vi "CODMn通讯.vi"() -> ()   [LabVIEW 2016, in "斯坦道CODMn.lvlib"]
uses:
  <vilib>/NI/Modbus Library/API/Wrapper/Create TCP Slave.vi
  <vilib>/NI/Modbus Library/API/slave/Modbus Slave.lvclass
  <vilib>/Plasmionique/MB Master/MB_Master/MB_Master.lvclass
  <vilib>/Plasmionique/MB Master/MB Master.lvlib
  <vilib>/Utility/config.llb/NI_LVConfig.lvlib
  <vilib>/NI/Modbus Library/API/Wrapper/API Main.lvlib
panel:
  in  "读取数据":bool
  in  "释放串口":bool
  in  "打开串口":bool
  out "队列中元素数量":i32
  out "元素":cluster{"命令":string}[](array[cluster])
  out "待处理插入数量":i32
  out "读取公式":u16[](array[numeric])
  out "读取参数":u16[](array[numeric])
  out "数据存储":u16[](array[numeric])
  out "温度":bool[](array[boolean])
  out "M输出点":bool[](array[boolean])
  out "ORP、时间":u16[](array[numeric])
  out "测量状态":u16[](array[numeric])
  out "通讯状态":bool
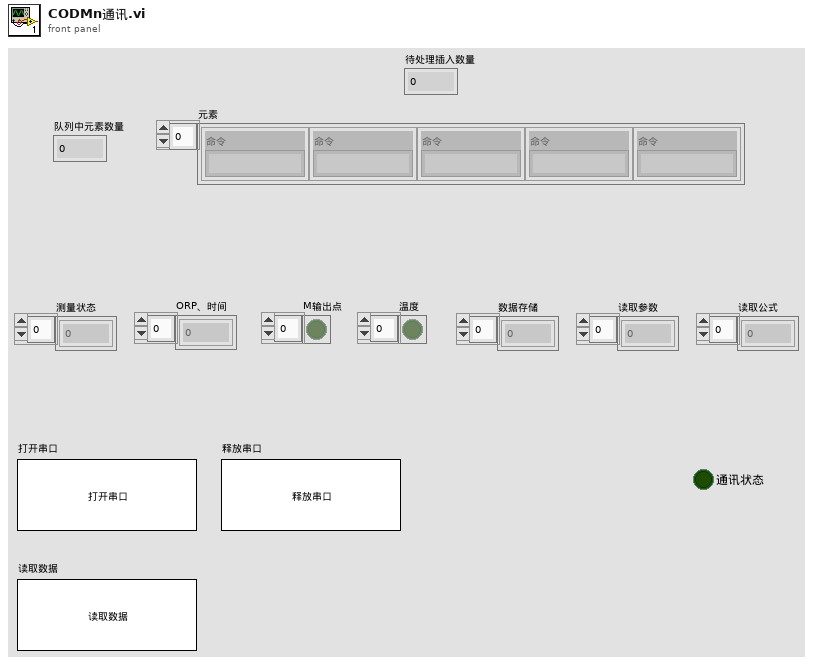
[diagram p1: front panel]
types:
  T1 = typedef "NI_LVConfig.lvlib/Config Data RefNum.ctl" = refnum<k1>
  T2 = enum16{"空闲", "水样测试", "标样核查", "零点核查", "跨度核查", "空白测试", "平行样测试", "质控样", "空白校准", "标样校准", "加标回收"}
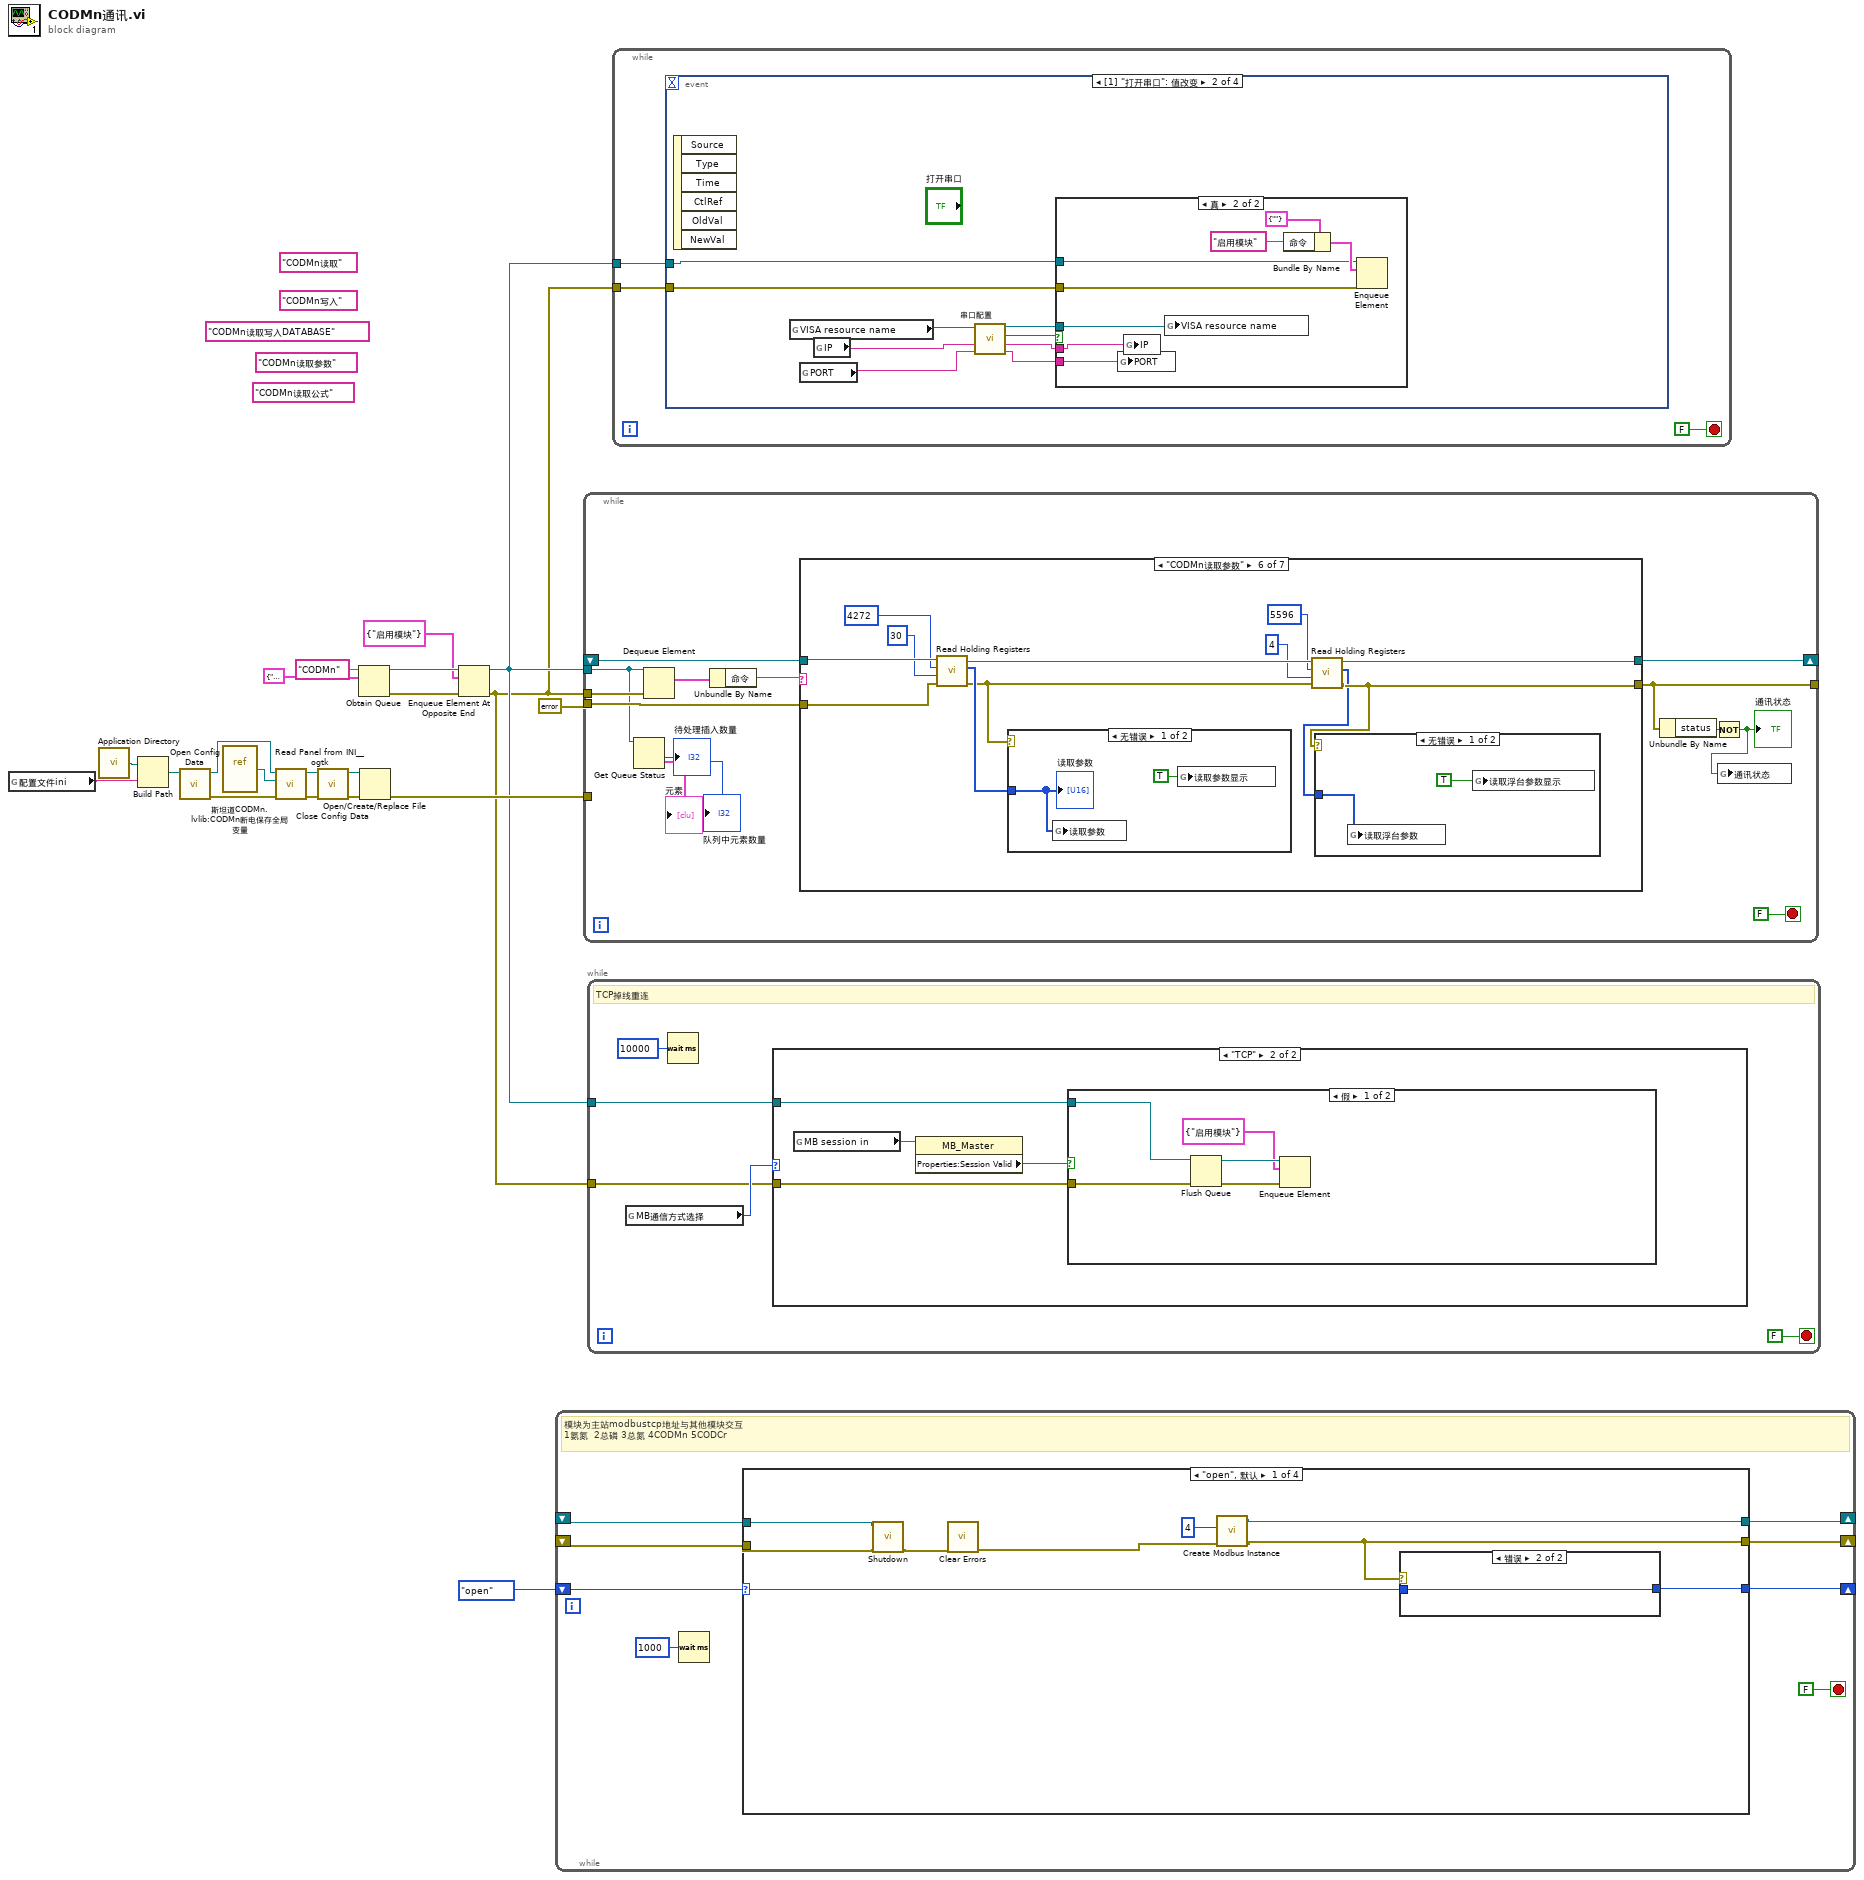
[diagram p0: block diagram]
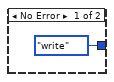
[diagram p4: hidden frame]
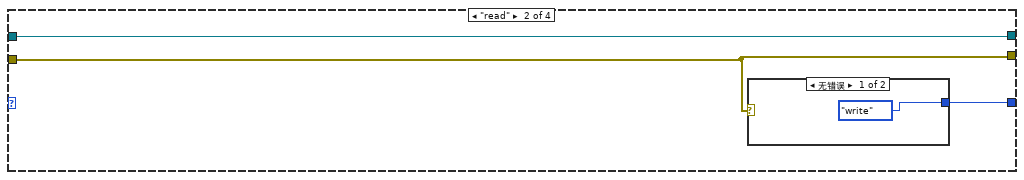
[diagram p5: hidden frame]
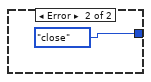
[diagram p6: hidden frame]
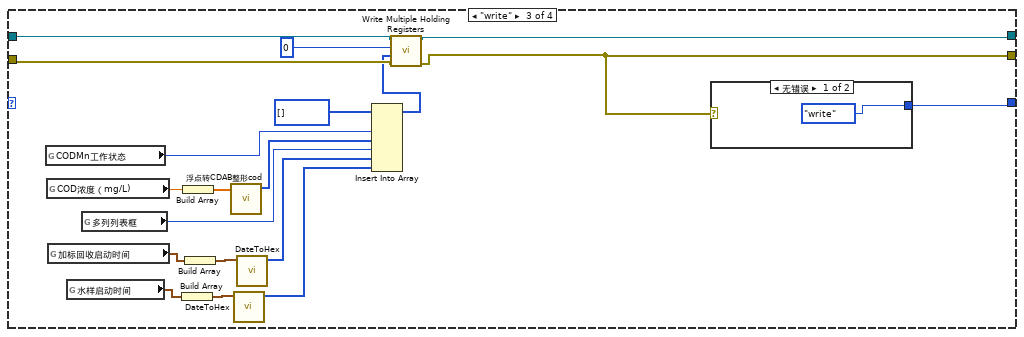
[diagram p7: hidden frame]
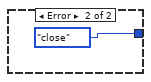
[diagram p8: hidden frame]
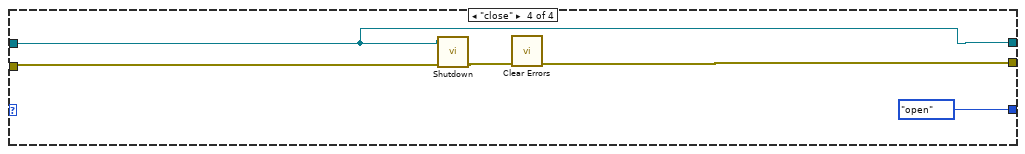
[diagram p9: hidden frame]
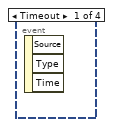
[diagram p10: hidden frame]
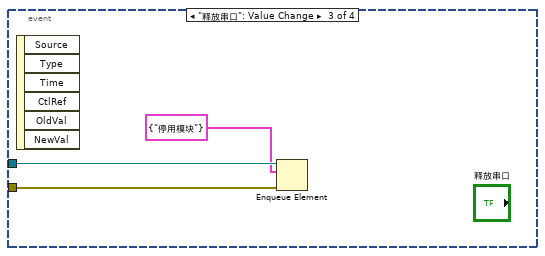
[diagram p12: hidden frame]
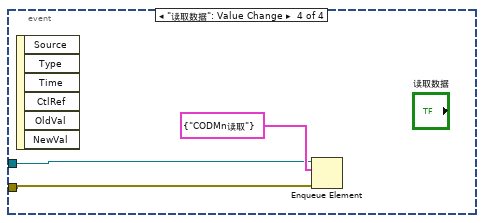
[diagram p13: hidden frame]
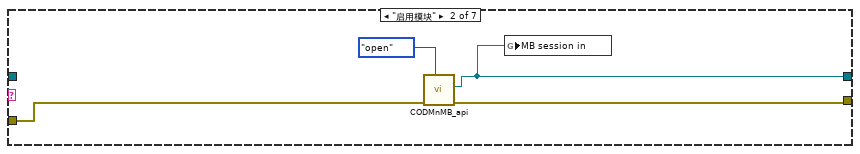
[diagram p15: hidden frame]
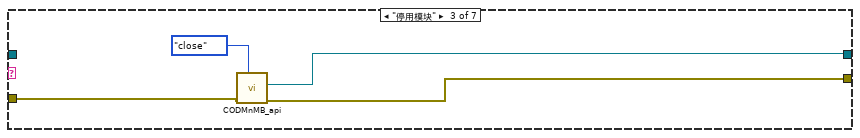
[diagram p16: hidden frame]
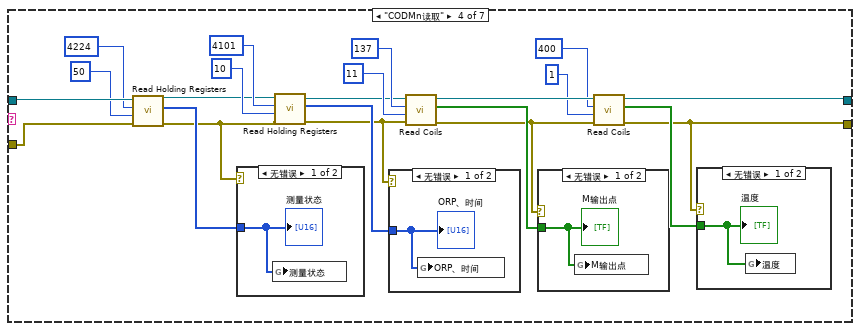
[diagram p17: hidden frame]
diagram:
  (unwired) "CODMn读取公式" ("名称（未命名）")
  (unwired) "CODMn读取写入DATABASE" ("名称（未命名）")
  (unwired) "CODMn读取参数" ("名称（未命名）")
  (unwired) "CODMn读取" ("名称（未命名）")
  (unwired) "CODMn写入" ("名称（未命名）")
  n1 = global read "COD读取DATA全局.vi" "配置文件ini"() -> (w1:string)
  n2 = call <vilib>:"Application Directory.vi"() -> ("Application Directory"=w14:path)
  n3 = Build Path(base path=w14, name or relative path=w1) -> (appended path=w13:path)
  n4 = call <vilib>:"Open Config Data.vi"("configuration file path"=w13) -> ("error out"=w9:errorcluster, "refnum"=w12:T1)  [unwired: 8 in, 1 out]
  n5 = vi-ref "斯坦道CODMn.lvlib:CODMn断电保存全局变量.vi"() -> (w11:refnum<vi>)
  n6 = call <userlib>:"Read Panel from INI__ogtk.vi"("error in (no error)"=w9, "VI ref"=w11, "refnum"=w12) -> ("error out"=w8:errorcluster, "refnum out"=w10:T1)  [unwired: 7 in]
  n7 = call <vilib>:"Close Config Data.vi"("error in (no error)"=w8, "refnum"=w10) -> ("error out"=w7:errorcluster, "file path"=w6:path)  [unwired: 8 in]
  n8 = Obtain Queue(name (unnamed)="CODMn" ("名称（未命名）"), element data type=cluster{"命令":string} {"命令"="启用模块"} ("元素")) -> (queue out=w17:refnum<queue>, error out=w16:errorcluster)  [unwired: 3 in, 1 out]
  n9 = Open/Create/Replace File(file path (use dialog)=w6, error in=w7) -> (error out=w5:errorcluster)  [unwired: 4 in, 2 out]
  n10 = Enqueue Element At Opposite End(queue=w17, element=cluster{"命令":string} {"命令"="启用模块"} ("元素"), error in (no error)=w16) -> (queue out=w3:refnum<queue>, error out=w2:errorcluster)  [unwired: 1 in, 1 out]
  n11 = while {
    shift-right: [w26] -> _
    shift-left: _ -> [w28]
    shift-right: [w25] -> _
    shift-left: _ -> [w27]
    shift-right: [w22] -> _
    shift-left: enum16{"open", "read", "write", "close"}."open" -> [w23]
    stop <- FALSE stop-if-true
    # "模块为主站modbustcp地址与其他模块交互\n1氨氮  2总磷 3总氮 4CODMn 5CODCr"
    n12 = Wait (ms)(milliseconds to wait=u32 1000 ("等待时间（毫秒）")) -> ()  [unwired: 1 out]
    n13 = case shown="\"open\", 默认" w23 {
      selector: w23 -> [w37 _ _ _]
      tunnel: w28 -> [w31 w40 w62 w68]
      tunnel: w27 -> [w30 w41 w59 w67]
      tunnel: [w34 w40 w61 w68] -> w26
      tunnel: [w33 w41 w60 w70] -> w25
      tunnel: [w36 w42 w63 enum16{"open", "read", "write", "close"}."open"] -> w22
      frame "open", Default {
        n14 = call-dynamic "Shutdown.vi"("error in"=w30, "Modbus slave in"=w31) -> ("error out"=w29:errorcluster)  [unwired: 9 in]
        n15 = call <vilib>:"Clear Errors.vi"("error in (no error)"=w29) -> ("error out"=w32:errorcluster)  [unwired: 5 in, 1 out]
        n16 = call-poly <vilib>:"Create Modbus Instance.vi"("error in"=w32, "port (502)"=u16 4) -> ("error out"=w33:errorcluster, "TCP slave instance"=w34:refnum<class "Modbus Slave.lvclass">)  [unwired: 8 in]
        n17 = case shown="错误" w33 {
          tunnel: w37 -> [_ w39]
          tunnel: [enum16{"open", "read", "write", "close"}."write" w39] -> w36
          frame No Error {
          }
          frame Error {
          }
        }
      }
      frame "read" {
        n18 = case shown="无错误" w41 {
          tunnel: [enum16{"open", "read", "write", "close"}."write" enum16{"open", "read", "write", "close"}."close"] -> w42
          frame No Error {
          }
          frame Error {
          }
        }
      }
      frame "write" {
        n19 = global read "COD测量模式全局.vi" "CODMn工作状态"() -> (w49:T2)
        n20 = global read "COD浓度全局变量.vi" "COD浓度（mg/L)"() -> (w51:dbl)
        n21 = global read "COD测量模式全局.vi" "加标回收启动时间"() -> (w54:timestamp)
        n22 = global read "COD测量模式全局.vi" "水样启动时间"() -> (w56:timestamp)
        n23 = global read "运行时序全局变量.vi" "多列列表框"() -> (w53:i32)
        n24 = Build Array(w56) -> (w55:timestamp[])
        n25 = Build Array(w51) -> (w50:dbl[])
        n26 = Build Array(w54) -> (w47:timestamp[])
        n27 = call "浮点转CDAB整形cod.vi"("浮点数"=w50) -> ("CDAB整形输出"=w52:u16[])  [unwired: 10 in]
        n28 = call "DateToHex.vi"("DATE"=w55) -> ("数组"=w58:u16[])  [unwired: 10 in]
        n29 = call "DateToHex.vi"("DATE"=w47) -> ("数组"=w57:u16[])  [unwired: 10 in]
        n30 = Insert Into Array(array=u16[] [] ("values"), new element #1=w49, new element #2=w52, new element #3=w53, new element #4=w57, new element #5=w58) -> (w46:u16[])  [unwired: 1 in]
        n31 = call-dynamic "Write Multiple Holding Registers.vi"("error in"=w59, "registers to write"=w46, "starting address"=u16 0, "Modbus slave in"=w62) -> ("error out"=w60:errorcluster, "Modbus slave out"=w61:refnum<class "Modbus Slave.lvclass">)  [unwired: 6 in]
        n32 = case shown="无错误" w60 {
          tunnel: [enum16{"open", "read", "write", "close"}."write" enum16{"open", "read", "write", "close"}."close"] -> w63
          frame No Error {
          }
          frame Error {
          }
        }
      }
      frame "close" {
        n33 = call-dynamic "Shutdown.vi"("error in"=w67, "Modbus slave in"=w68) -> ("error out"=w66:errorcluster)  [unwired: 9 in]
        n34 = call <vilib>:"Clear Errors.vi"("error in (no error)"=w66) -> ("error out"=w70:errorcluster)  [unwired: 5 in, 1 out]
      }
    }
  }
  n35 = while {
    tunnel: w3 -> [w74]
    tunnel: w2 -> [w83]
    tunnel: [w75] -> _
    shift-right: [w79] -> _
    shift-left: _ -> [w78]
    tunnel: errorcluster {"status"=FALSE, "code"=0, "source"=""} ("error out") -> [w77]
    tunnel: w5 -> [_]
    stop <- FALSE stop-if-true
    n36 = Get Queue Status(queue=w74) -> (# pending insert=→"待处理插入数量":i32, # elements in queue=→"队列中元素数量":i32, elements=→"元素":cluster{"命令":string}[])  [unwired: 2 in, 5 out]
    n37 = Dequeue Element(queue=w74, error in (no error)=w83) -> (element=w82:cluster{"命令":string})  [unwired: 1 in, 3 out]
    n38 = Unbundle By Name(w82) -> ("命令"=w81:string)
    n39 = case shown="\"CODMn读取参数\"" w81 {
      tunnel: [w86 w87 w91 w102 w123 w132 w149] -> w79
      tunnel: [w85 w90 w92 w95 w121 w131 w148] -> w75
      tunnel: w78 -> [w86 _ _ w116 w127 w141 w152]
      tunnel: w77 -> [w85 w88 w93 w115 w124 w140 w151]
      frame Default {
      }
      frame "启用模块" {
        n40 = call "CODMnMB_api.vi"("STEP"=enum16{"open", "read", "write", "close"}."open", "Error in"=w88) -> ("error out"=w90:errorcluster, "MB session out"=w87:refnum<class "MB_Master.lvclass">)  [unwired: 7 in, 1 out]
        n41 = global write "COD浓度全局变量.vi" "MB session in"(w87) -> ()
      }
      frame "停用模块" {
        n42 = call "CODMnMB_api.vi"("STEP"=enum16{"open", "read", "write", "close"}."close", "Error in"=w93) -> ("error out"=w92:errorcluster, "MB session out"=w91:refnum<class "MB_Master.lvclass">)  [unwired: 7 in, 1 out]
      }
      frame "CODMn读取" {
        n43 = call <vilib>:"Read Holding Registers.vi"("error in (no error)"=w115, "quantity"=u16 50 ("number of holding registers"), "starting address"=u16 4224, "MB session in"=w116) -> ("error out"=w106:errorcluster, "Registers"=w112:u16[], "MB session out"=w107:refnum<class "MB_Master.lvclass">)  [unwired: 5 in]
        n44 = case shown="无错误" w106 {
          tunnel: w112 -> [w120 _]
          frame No Error {
            n45 = global write "COD读取DATA全局.vi" "测量状态"(w120) -> ()
            "测量状态" <- w120
          }
          frame Error {
          }
        }
        n46 = call <vilib>:"Read Holding Registers.vi"("error in (no error)"=w106, "quantity"=u16 10, "starting address"=u16 4101, "MB session in"=w107) -> ("error out"=w101:errorcluster, "Registers"=w105:u16[], "MB session out"=w104:refnum<class "MB_Master.lvclass">)  [unwired: 5 in]
        n47 = case shown="无错误" w101 {
          tunnel: w105 -> [w119 _]
          frame No Error {
            n48 = global write "COD读取DATA全局.vi" "ORP、时间"(w119) -> ()
            "ORP、时间" <- w119
          }
          frame Error {
          }
        }
        n49 = call <vilib>:"Read Coils.vi"("error in (no error)"=w101, "quantity"=u16 11, "starting address"=u16 137, "MB session in"=w104) -> ("error out"=w99:errorcluster, "Coils"=w100:bool[], "MB session out"=w103:refnum<class "MB_Master.lvclass">)  [unwired: 5 in]
        n50 = case shown="无错误" w99 {
          tunnel: w100 -> [w118 _]
          frame No Error {
            n51 = global write "COD读取DATA全局.vi" "M输出点"(w118) -> ()
            "M输出点" <- w118
          }
          frame Error {
          }
        }
        n52 = call <vilib>:"Read Coils.vi"("error in (no error)"=w99, "quantity"=u16 1, "starting address"=u16 400, "MB session in"=w103) -> ("error out"=w95:errorcluster, "Coils"=w96:bool[], "MB session out"=w102:refnum<class "MB_Master.lvclass">)  [unwired: 5 in]
        n53 = case shown="无错误" w95 {
          tunnel: w96 -> [w117 _]
          frame No Error {
            n54 = global write "COD读取DATA全局.vi" "温度"(w117) -> ()
            "温度" <- w117
          }
          frame Error {
          }
        }
      }
      frame "CODMn读取写入DATABASE" {
        n55 = call <vilib>:"Read Holding Registers.vi"("error in (no error)"=w124, "quantity"=u16 10 ("number of holding registers"), "starting address"=u16 4101, "MB session in"=w127) -> ("error out"=w121:errorcluster, "Registers"=w122:u16[], "MB session out"=w123:refnum<class "MB_Master.lvclass">)  [unwired: 5 in]
        n56 = case shown="无错误" w121 {
          tunnel: w122 -> [w129 _]
          frame No Error {
            n57 = global write "COD读取DATA全局.vi" "数据存储"(w129) -> ()
            n58 = global write "COD读取DATA全局.vi" "读取写入data"(TRUE ("读取参数显示")) -> ()
            "数据存储" <- w129
          }
          frame Error {
          }
        }
      }
      frame "CODMn读取参数" {
        n59 = call <vilib>:"Read Holding Registers.vi"("error in (no error)"=w140, "quantity"=u16 30 ("number of holding registers"), "starting address"=u16 4272, "MB session in"=w141) -> ("error out"=w135:errorcluster, "Registers"=w137:u16[], "MB session out"=w136:refnum<class "MB_Master.lvclass">)  [unwired: 5 in]
        n60 = case shown="无错误" w135 {
          tunnel: w137 -> [w145 _]
          frame No Error {
            n61 = global write "COD读取DATA全局.vi" "读取参数"(w145) -> ()
            n62 = global write "COD读取DATA全局.vi" "读取参数显示"(TRUE ("读取参数显示")) -> ()
            "读取参数" <- w145
          }
          frame Error {
          }
        }
        n63 = call <vilib>:"Read Holding Registers.vi"("error in (no error)"=w135, "quantity"=u16 4, "starting address"=u16 5596, "MB session in"=w136) -> ("error out"=w131:errorcluster, "Registers"=w130:u16[], "MB session out"=w132:refnum<class "MB_Master.lvclass">)  [unwired: 5 in]
        n64 = case shown="无错误" w131 {
          tunnel: w130 -> [w143 _]
          frame No Error {
            n65 = global write "COD读取DATA全局.vi" "读取浮台参数"(w143) -> ()
            n66 = global write "COD读取DATA全局.vi" "读取浮台参数显示"(TRUE ("读取参数显示")) -> ()
          }
          frame Error {
          }
        }
      }
      frame "CODMn读取公式" {
        n67 = call <vilib>:"Read Holding Registers.vi"("error in (no error)"=w151, "quantity"=u16 94 ("number of holding registers"), "starting address"=u16 4616, "MB session in"=w152) -> ("error out"=w148:errorcluster, "Registers"=w150:u16[], "MB session out"=w149:refnum<class "MB_Master.lvclass">)  [unwired: 5 in]
        n68 = case shown="无错误" w148 {
          tunnel: w150 -> [w154 _]
          frame No Error {
            n69 = global write "COD读取DATA全局.vi" "读取公式"(w154) -> ()
            n70 = global write "COD读取DATA全局.vi" "读取公式显示"(TRUE ("读取参数显示")) -> ()
            "读取公式" <- w154
          }
          frame Error {
          }
        }
      }
    }
    n71 = Unbundle By Name(w75) -> ("status"=w80:bool)
    n72 = Not(x=w80) -> (.not. x?=w76:bool)
    "通讯状态" <- w76
    n73 = global write "COD读取DATA全局.vi" "通讯状态"(w76) -> ()
  }
  n74 = while "While循环" {
    tunnel: w3 -> [w156]
    tunnel: w2 -> [w155]
    stop <- FALSE stop-if-true
    # "TCP掉线重连"
    n75 = global read "CODMn断电保存全局变量.vi" "MB通信方式选择"() -> (w157:enum16{"串口", "TCP"})
    n76 = Wait (ms)(milliseconds to wait=u32 10000 ("等待时间（毫秒）")) -> ()  [unwired: 1 out]
    n77 = case shown="\"TCP\"" w157 {
      tunnel: w156 -> [_ w161]
      tunnel: w155 -> [_ w160]
      frame "串口", Default {
      }
      frame "TCP" {
        n78 = global read "COD浓度全局变量.vi" "MB session in"() -> (w163:refnum<class "MB_Master.lvclass">)
        n79 = property class="MB_Master"(reference=w163) -> ("Properties:Session Valid"=w162:bool)  [unwired: 1 in, 2 out]
        n80 = case shown="假" w162 {
          tunnel: w161 -> [w165 _]
          tunnel: w160 -> [w164 _]
          frame False {
            n81 = Flush Queue(queue=w165, error in (no error)=w164) -> (queue out=w168:refnum<queue>, error out=w167:errorcluster)  [unwired: 1 out]
            n82 = Enqueue Element(queue=w168, element=cluster{"命令":string} {"命令"="启用模块"} ("元素"), error in (no error)=w167) -> ()  [unwired: 1 in, 3 out]
          }
          frame True {
          }
        }
      }
    }
  }
  n83 = while {
    tunnel: w3 -> [w170]
    tunnel: w2 -> [w169]
    stop <- FALSE stop-if-true
    n84 = event shown="[1] \"打开串口\": 值改变" {
      selector: _ -> [_ _ _ _]
      dyn-events: _ -> [_ _ _ _]
      timeout: _ -> [_ _ _ _]
      tunnel: w170 -> [_ w177 w191 w193]
      tunnel: w169 -> [_ w176 w190 w192]
      event Timeout {
        n85 = event-data() -> ()  [unwired: 1 in, 3 out]
      }
      event "打开串口": Value Change {
        n86 = event-data() -> ()  [unwired: 1 in, 6 out]
        n87 = global read "CODMn断电保存全局变量.vi" "VISA resource name"() -> (w180:refnum<visa-resource-name>)
        n88 = global read "CODMn断电保存全局变量.vi" "PORT"() -> (w172:string)
        n89 = global read "CODMn断电保存全局变量.vi" "IP"() -> (w173:string)
        n90 = call "串口配置.vi"("PORT"=w172, "IP"=w173, "请选择串口:"=w180) -> ("PORT 2"=w174:string, "IP 2"=w175:string, "确认 2"=w178:bool, "VISA资源名称 2"=w179:refnum<visa-resource-name>)  [unwired: 4 in, 1 out]
        n91 = case shown="真" w178 {
          tunnel: w179 -> [_ w188]
          tunnel: w177 -> [_ w184]
          tunnel: w176 -> [_ w183]
          tunnel: w175 -> [_ w182]
          tunnel: w174 -> [_ w181]
          frame False {
          }
          frame True {
            n92 = global write "CODMn断电保存全局变量.vi" "PORT"(w181) -> ()
            n93 = global write "CODMn断电保存全局变量.vi" "IP"(w182) -> ()
            n94 = global write "CODMn断电保存全局变量.vi" "VISA resource name"(w188) -> ()
            n95 = Bundle By Name(cluster=cluster{"命令":string} {"命令"=""} ("元素"), "命令"="启用模块" ("名称（未命名）")) -> (w185:cluster{"命令":string})
            n96 = Enqueue Element(queue=w184, element=w185, error in (no error)=w183) -> ()  [unwired: 1 in, 3 out]
          }
        }
      }
      event "释放串口": Value Change {
        n97 = event-data() -> ()  [unwired: 1 in, 6 out]
        n98 = Enqueue Element(queue=w191, element=cluster{"命令":string} {"命令"="停用模块"} ("元素"), error in (no error)=w190) -> ()  [unwired: 1 in, 3 out]
      }
      event "读取数据": Value Change {
        n99 = event-data() -> ()  [unwired: 1 in, 6 out]
        n100 = Enqueue Element(queue=w193, element=cluster{"命令":string} {"命令"="CODMn读取"} ("元素"), error in (no error)=w192) -> ()  [unwired: 1 in, 3 out]
      }
    }
  }
